vi "Calculate Channel Voltage.vi"(7 "Scale":i32, 8 "error in (no error)":errorcluster, 9 "ChanSpanOffset":i32, 10 "ChanZeroOffset":i32, 11 "ChanValue":i32) -> (0 "error out":errorcluster, 3 "Channel Voltage Result":dbl)   [LabVIEW 2015]
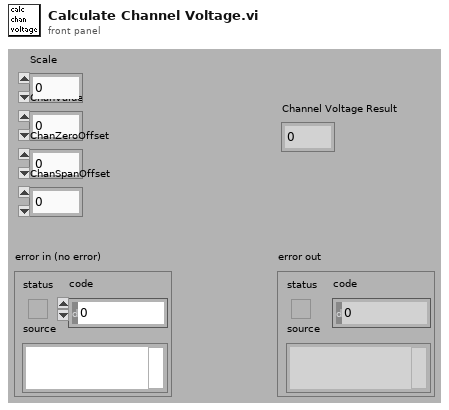
[diagram p1: front panel]
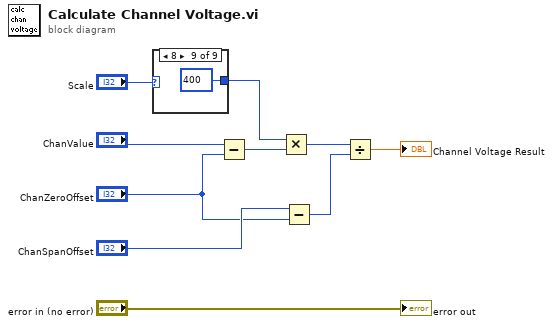
[diagram p0: block diagram]
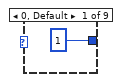
[diagram p2: hidden frame]
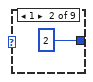
[diagram p3: hidden frame]
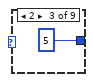
[diagram p4: hidden frame]
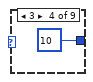
[diagram p5: hidden frame]
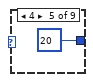
[diagram p6: hidden frame]
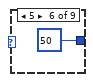
[diagram p7: hidden frame]
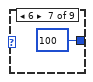
[diagram p8: hidden frame]
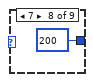
[diagram p9: hidden frame]
diagram:
  n1 = case shown="8" "Scale" {
    tunnel: [1 2 5 10 20 50 100 200 400] -> w1
    frame 0, Default {
    }
    frame 1 {
    }
    frame 2 {
    }
    frame 3 {
    }
    frame 4 {
    }
    frame 5 {
    }
    frame 6 {
    }
    frame 7 {
    }
    frame 8 {
    }
  }
  n2 = Subtract(x="ChanValue", y="ChanZeroOffset") -> (x-y=w8:i32)
  n3 = Multiply(x=w1, y=w8) -> (x*y=w7:i32)
  n4 = Subtract(x="ChanSpanOffset", y="ChanZeroOffset") -> (x-y=w4:i32)
  n5 = Divide(x=w7, y=w4) -> (x/y=→"Channel Voltage Result":dbl)
  "error out" <- "error in (no error)"
